vi "write_phase.vi"(6 "Filename":string, 7 "Default filename":string, 9 "Array":dbl[][](array[numeric]), 10 "format (%.3f)":string, 11 "Phase folder":path) -> (0 "error out":errorcluster, 2 "error?":bool, 3 "new file path (Not A Path if cancelled)":path)   [LabVIEW 2022 SP3]
uses:
  <vilib>/Utility/file.llb/Write Delimited Spreadsheet (DBL).vi
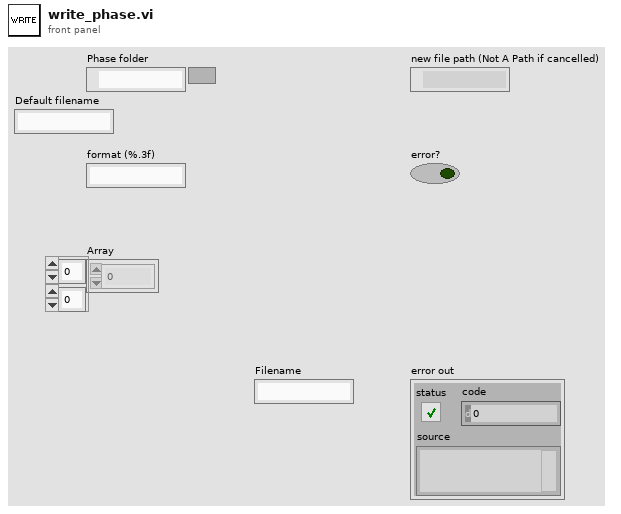
[diagram p1: front panel]
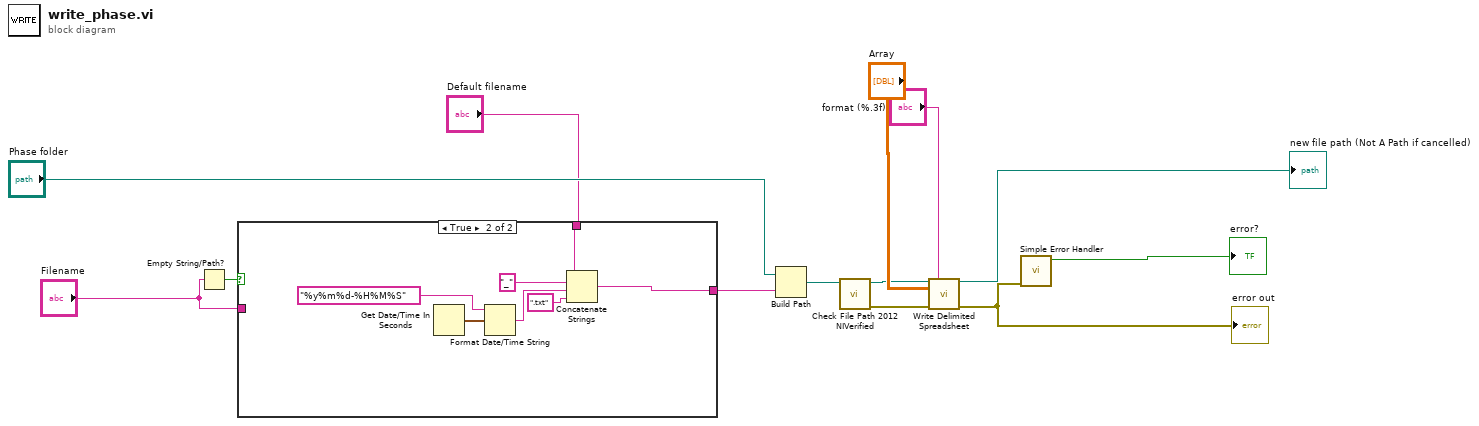
[diagram p0: block diagram]
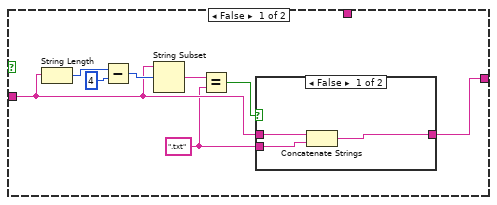
[diagram p2: hidden frame]
diagram:
  n1 = Empty String/Path?(string/path="Filename") -> (empty?=w3:bool)
  n2 = case shown="True" w3 {
    tunnel: "Filename" -> [w16 _]
    tunnel: [w15 w28] -> w4
    tunnel: "Default filename" -> [_ w26]
    frame False {
      w14 = ".txt" ("y")
      n3 = String Length(string=w16) -> (length=w20:i32)
      n4 = Subtract(x=w20, y=4) -> (x-y=w21:i32)
      n5 = String Subset(string=w16, offset (0)=w21) -> (substring=w18:string)  [unwired: 1 in]
      n6 = Equal?(x=w18, y=w14) -> (x = y?=w17:bool)
      n7 = case shown="False" w17 {
        tunnel: [w23 w25] -> w15
        tunnel: w16 -> [w24 w25]
        tunnel: w14 -> [w22 _]
        frame False {
          n8 = Concatenate Strings(w24, w22) -> (w23:string)
        }
        frame True {
        }
      }
    }
    frame True {
      n9 = Get Date/Time In Seconds() -> (seconds since 1Jan1904=w32:timestamp)
      n10 = Format Date/Time String(time format string (%c)="%y%m%d-%H%M%S", seconds (now)=w32) -> (date/time string=w30:string)  [unwired: 1 in]
      n11 = Concatenate Strings(w26, "_" ("string"), w30, ".txt" ("string")) -> (w28:string)
    }
  }
  n12 = Build Path(base path="Phase folder", name or relative path=w4) -> (appended path=w6:path)
  n13 = call "Check File Path 2012 NIVerified.vi"("Path to Check"=w6) -> ("error out"=w10:errorcluster, "Valid Path"=w7:path)  [unwired: 7 in, 2 out]
  n14 = call-poly <vilib>:"Write Delimited Spreadsheet.vi"("file path (dialog if empty)"=w7, "format (%.3f)"="format (%.3f)", "2D data"="Array", "error in (no error)"=w10) -> ("new file path (Not A Path if cancelled)"=→"new file path (Not A Path if cancelled)":path, "error out"=w11:errorcluster)  [unwired: 10 in]
  "error out" <- w11
  n15 = call <vilib>:"Simple Error Handler.vi"("error in (no error)"=w11) -> ("error?"=→"error?":bool)  [unwired: 4 in, 4 out]
